vi "Plugin - Sine Graph.vi"() -> ()   [LabVIEW 2014]
doc: "正弦波を様々な位相で波形グラフ上に表示するサブパネルプラグインVI。"
panel:
  in  "パラメータ":string[](array[string])
  out "波形グラフ":dynamicdata(graph)
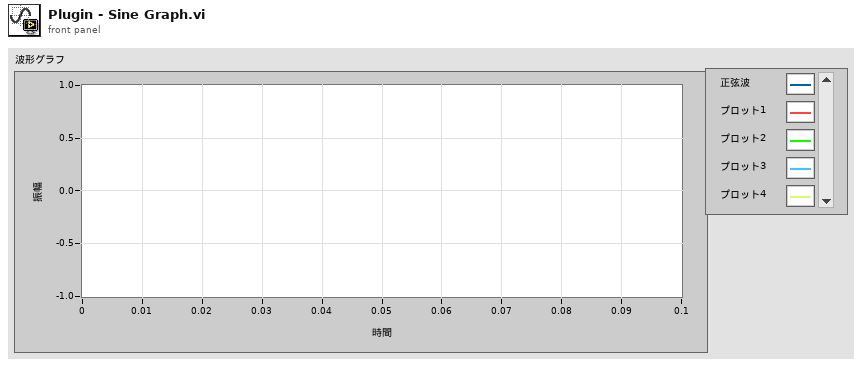
[diagram p1: front panel]
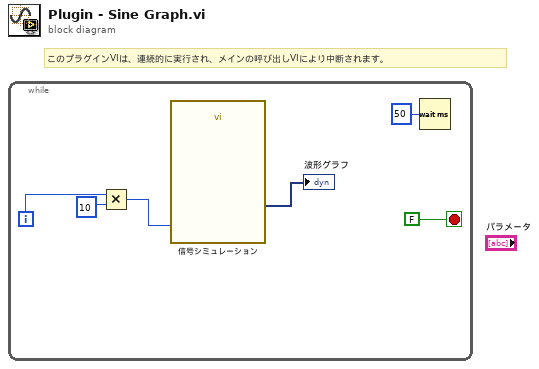
[diagram p0: block diagram]
diagram:
  # "このプラグインVIは、連続的に実行され、メインの呼び出しVIにより中断されます。"
  n1 = while {
    i -> [w5]
    stop <- FALSE stop-if-true
    n2 = Multiply(x=w5, y=10) -> (x*y=w1:i32)
    n3 = call "信号シミュレーション"("Phase"=w1) -> ("Sine"=→"波形グラフ":dynamicdata)  [unwired: 13 in, 1 out]
    n4 = Wait (ms)(milliseconds to wait=u32 50) -> ()  [unwired: 1 out]
  }
